vi "RW_setV.vi"(8 "error in (no error)":errorcluster, 10 "voltage":dbl, 11 "VISAsession":refnum<visa-resource-name>="wavefactoryU5") -> (0 "error out":errorcluster caption="Error OUT")   [LabVIEW 2018]
panel:
  out "elapsed time (ms)":u32=246
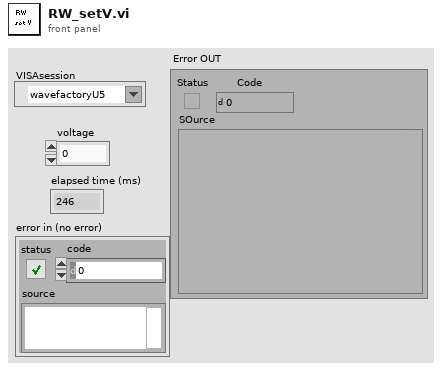
[diagram p1: front panel]
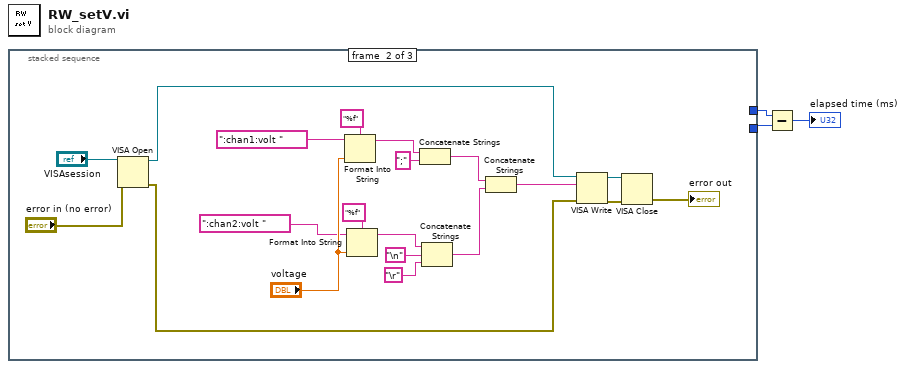
[diagram p0: block diagram]
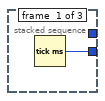
[diagram p2: hidden frame]
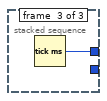
[diagram p3: hidden frame]
diagram:
  n1 = stacked-sequence {
    tunnel: [w4 _ _] -> w2
    tunnel: [_ _ w25] -> w3
    frame #0 {
      n2 = Tick Count (ms)() -> (millisecond timer value=w4:u32)
    }
    frame #1 {
      n3 = VISA Open(error in (no error)="error in (no error)", VISA resource name="VISAsession") -> (VISA resource name=w13:refnum<visa-resource-name>, error out=w14:errorcluster)  [unwired: 3 in]
      n4 = Format Into String(format string="%f", initial string=":chan1:volt ", "voltage") -> (resulting string=w24:string)  [unwired: 1 in, 1 out]
      n5 = Format Into String(format string="%f", initial string=":chan2:volt ", "voltage") -> (resulting string=w20:string)  [unwired: 1 in, 1 out]
      n6 = Concatenate Strings(w24, ";" ("string")) -> (w6:string)
      n7 = Concatenate Strings(w20, "\n", "\r") -> (w17:string)
      n8 = Concatenate Strings(w6, w17) -> (w5:string)
      n9 = VISA Write(VISA resource name=w13, write buffer=w5, error in (no error)=w14) -> (VISA resource name out=w16:refnum<visa-resource-name>, error out=w15:errorcluster)  [unwired: 1 out]
      n10 = VISA Close(VISA resource name=w16, error in (no error)=w15) -> (error out=→"error out":errorcluster)
    }
    frame #2 {
      n11 = Tick Count (ms)() -> (millisecond timer value=w25:u32)
    }
  }
  n12 = Subtract(x=w3, y=w2) -> (x-y=→"elapsed time (ms)":u32)
